vi "#1_MAV_MSG_SYS_STATUS_DECODE.vi"(11 "mavlink_payload":u8[](array[numeric])) -> (3 "SYS_STATUS":T1)   [LabVIEW 2023]
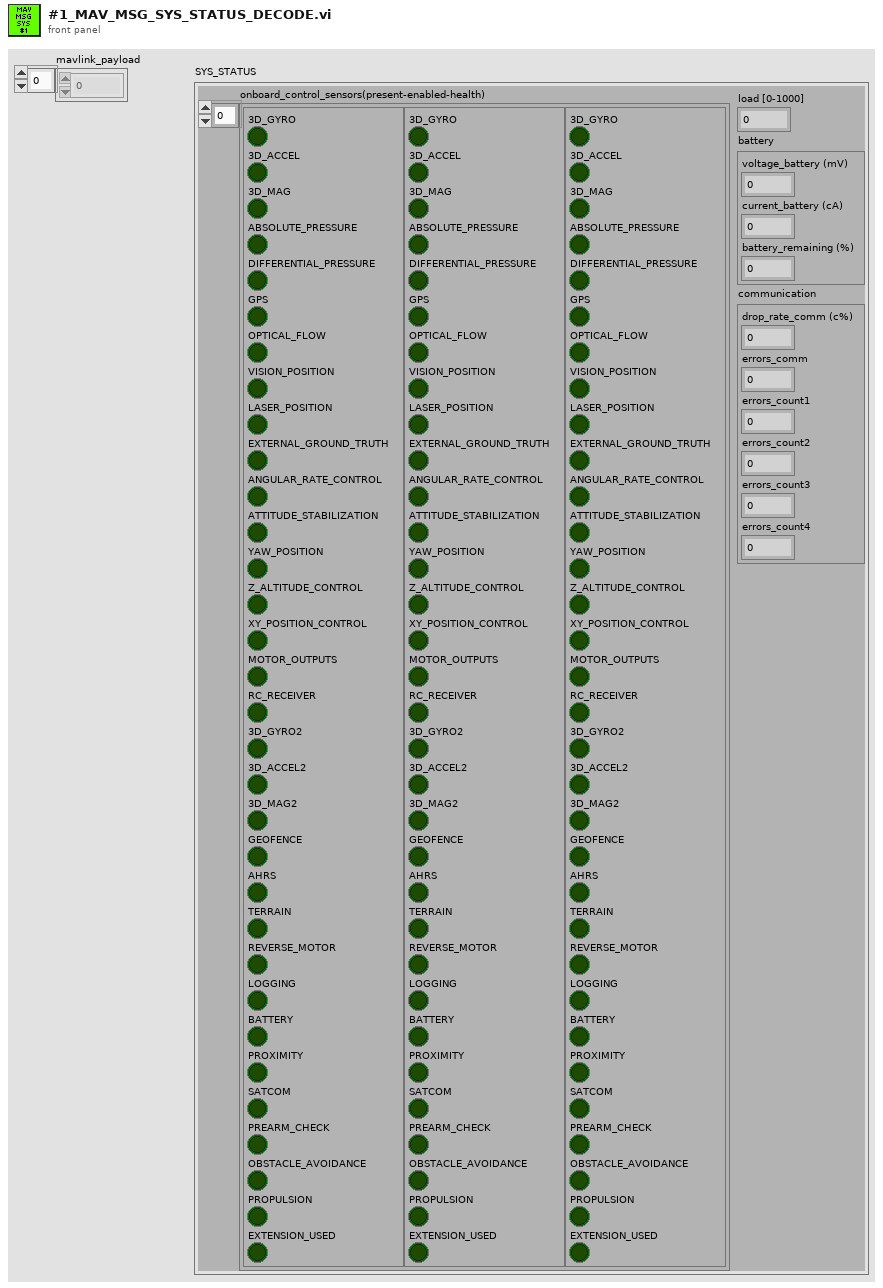
[diagram p1: front panel]
types:
  T1 = cluster{"onboard_control_sensors(present-enabled-health)":cluster{"3D_GYRO":bool, "3D_ACCEL":bool, "3D_MAG":bool, "ABSOLUTE_PRESSURE":bool, "DIFFERENTIAL_PRESSURE":bool, "GPS":bool, "OPTICAL_FLOW":bool, "VISION_POSITION":bool, "LASER_POSITION":bool, "EXTERNAL_GROUND_TRUTH":bool, "ANGULAR_RATE_CONTROL":bool, "ATTITUDE_STABILIZATION":bool, "YAW_POSITION":bool, "Z_ALTITUDE_CONTROL":bool, "XY_POSITION_CONTROL":bool, "MOTOR_OUTPUTS":bool, "RC_RECEIVER":bool, "3D_GYRO2":bool, "3D_ACCEL2":bool, "3D_MAG2":bool, "GEOFENCE":bool, "AHRS":bool, "TERRAIN":bool, "REVERSE_MOTOR":bool, "LOGGING":bool, "BATTERY":bool, "PROXIMITY":bool, "SATCOM":bool, "PREARM_CHECK":bool, "OBSTACLE_AVOIDANCE":bool, "PROPULSION":bool, "EXTENSION_USED":bool}[], "load [0-1000]":u16, "battery":cluster{"voltage_battery (mV)":u16, "current_battery (cA)":i16, "battery_remaining (%)":i8}, "communication":cluster{"drop_rate_comm (c%)":u16, "errors_comm":u16, "errors_count1":u16, "errors_count2":u16, "errors_count3":u16, "errors_count4":u16}}
  T2 = cluster{"drop_rate_comm (c%)":u16, "errors_comm":u16, "errors_count1":u16, "errors_count2":u16, "errors_count3":u16, "errors_count4":u16}
  T3 = cluster{"voltage_battery (mV)":u16, "current_battery (cA)":i16, "battery_remaining (%)":i8}
  T4 = cluster{"3D_GYRO":bool, "3D_ACCEL":bool, "3D_MAG":bool, "ABSOLUTE_PRESSURE":bool, "DIFFERENTIAL_PRESSURE":bool, "GPS":bool, "OPTICAL_FLOW":bool, "VISION_POSITION":bool, "LASER_POSITION":bool, "EXTERNAL_GROUND_TRUTH":bool, "ANGULAR_RATE_CONTROL":bool, "ATTITUDE_STABILIZATION":bool, "YAW_POSITION":bool, "Z_ALTITUDE_CONTROL":bool, "XY_POSITION_CONTROL":bool, "MOTOR_OUTPUTS":bool, "RC_RECEIVER":bool, "3D_GYRO2":bool, "3D_ACCEL2":bool, "3D_MAG2":bool, "GEOFENCE":bool, "AHRS":bool, "TERRAIN":bool, "REVERSE_MOTOR":bool, "LOGGING":bool, "BATTERY":bool, "PROXIMITY":bool, "SATCOM":bool, "PREARM_CHECK":bool, "OBSTACLE_AVOIDANCE":bool, "PROPULSION":bool, "EXTENSION_USED":bool}[]
  T5 = cluster{"Boolean array[0]":bool, "Boolean array[1]":bool, "Boolean array[2]":bool, "Boolean array[3]":bool, "Boolean array[4]":bool, "Boolean array[5]":bool, "Boolean array[6]":bool, "Boolean array[7]":bool, "Boolean array[8]":bool, "Boolean array[9]":bool, "Boolean array[10]":bool, "Boolean array[11]":bool, "Boolean array[12]":bool, "Boolean array[13]":bool, "Boolean array[14]":bool, "Boolean array[15]":bool, "Boolean array[16]":bool, "Boolean array[17]":bool, "Boolean array[18]":bool, "Boolean array[19]":bool, "Boolean array[20]":bool, "Boolean array[21]":bool, "Boolean array[22]":bool, "Boolean array[23]":bool, "Boolean array[24]":bool, "Boolean array[25]":bool, "Boolean array[26]":bool, "Boolean array[27]":bool, "Boolean array[28]":bool, "Boolean array[29]":bool, "Boolean array[30]":bool, "Boolean array[31]":bool}
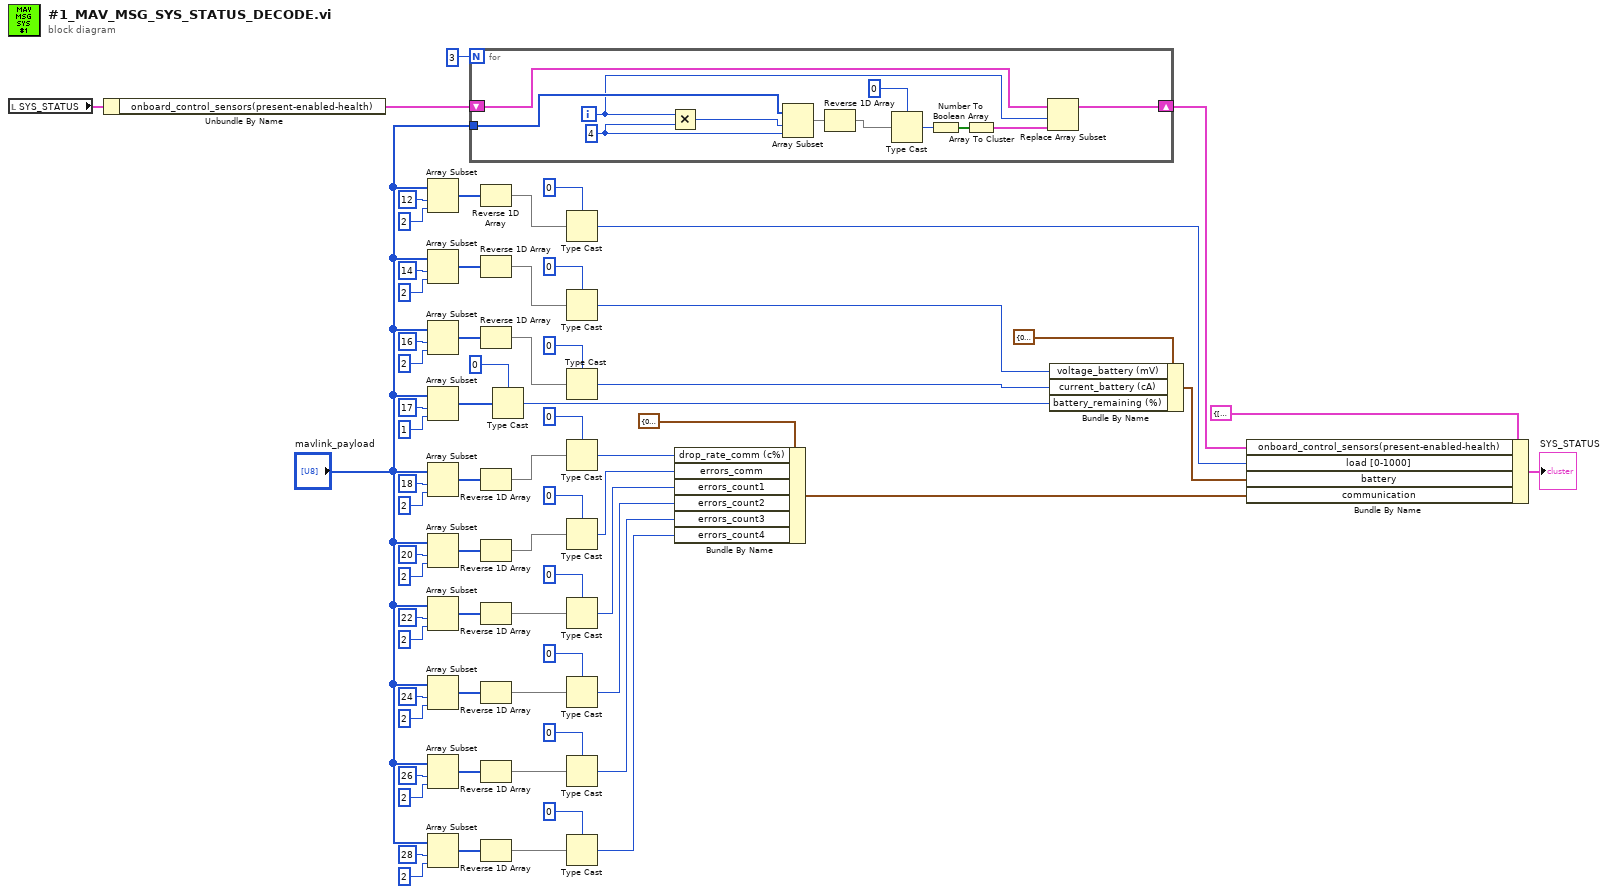
[diagram p0: block diagram]
diagram:
  n1 = local read "SYS_STATUS"() -> (w63:T1)
  n2 = Unbundle By Name(w63) -> ("onboard_control_sensors(present-enabled-health)"=w62:T4)
  n3 = Array Subset(array="mavlink_payload", index=12, length=2) -> (w65:u8[])
  n4 = Array Subset(array="mavlink_payload", index=14, length=2) -> (w60:u8[])
  n5 = Array Subset(array="mavlink_payload", index=16, length=2) -> (w50:u8[])
  n6 = Array Subset(array="mavlink_payload", index=17, length=1) -> (w41:u8[])
  n7 = Array Subset(array="mavlink_payload", index=18, length=2) -> (w38:u8[])
  n8 = Array Subset(array="mavlink_payload", index=20, length=2) -> (w30:u8[])
  n9 = Array Subset(array="mavlink_payload", index=22, length=2) -> (w24:u8[])
  n10 = Array Subset(array="mavlink_payload", index=24, length=2) -> (w19:u8[])
  n11 = Array Subset(array="mavlink_payload", index=26, length=2) -> (w12:u8[])
  n12 = Array Subset(array="mavlink_payload", index=28, length=2) -> (w7:u8[])
  n13 = for {
    N: 3 -> [_]
    tunnel: "mavlink_payload" -> [w78]
    shift-right: [w77] -> w64
    shift-left: w62 -> [w76]
    i -> [w74]
    w75 = 4 ("length")
    n14 = Multiply(x=w74, y=w75) -> (x*y=w73:i32)
    n15 = Array Subset(array=w78, index=w73, length=w75) -> (w80:u8[])
    n16 = Reverse 1D Array(array=w80) -> (reversed array=w81:u8[])
    n17 = Type Cast(type=u32 0, x=w81) -> (*(type *) &x=w82:u32)
    n18 = Number To Boolean Array(number=w82) -> (Boolean array=w72:bool[])
    n19 = Array To Cluster(array=w72) -> (cluster=w71:T5)
    n20 = Replace Array Subset(array=w76, new element=w71, index=w74) -> (w77:T4)
  }
  n21 = Reverse 1D Array(array=w65) -> (reversed array=w67:u8[])
  n22 = Reverse 1D Array(array=w60) -> (reversed array=w61:u8[])
  n23 = Reverse 1D Array(array=w50) -> (reversed array=w51:u8[])
  n24 = Reverse 1D Array(array=w38) -> (reversed array=w39:u8[])
  n25 = Reverse 1D Array(array=w30) -> (reversed array=w31:u8[])
  n26 = Reverse 1D Array(array=w24) -> (reversed array=w25:u8[])
  n27 = Reverse 1D Array(array=w19) -> (reversed array=w20:u8[])
  n28 = Reverse 1D Array(array=w12) -> (reversed array=w13:u8[])
  n29 = Reverse 1D Array(array=w7) -> (reversed array=w8:u8[])
  n30 = Type Cast(type=i8 0, x=w41) -> (*(type *) &x=w40:i8)
  n31 = Type Cast(type=u16 0, x=w67) -> (*(type *) &x=w59:u16)
  n32 = Type Cast(type=u16 0, x=w61) -> (*(type *) &x=w52:u16)
  n33 = Type Cast(type=i16 0, x=w51) -> (*(type *) &x=w47:i16)
  n34 = Type Cast(type=u16 0, x=w39) -> (*(type *) &x=w32:u16)
  n35 = Type Cast(type=u16 0, x=w31) -> (*(type *) &x=w26:u16)
  n36 = Type Cast(type=u16 0, x=w25) -> (*(type *) &x=w15:u16)
  n37 = Type Cast(type=u16 0, x=w20) -> (*(type *) &x=w14:u16)
  n38 = Type Cast(type=u16 0, x=w13) -> (*(type *) &x=w2:u16)
  n39 = Type Cast(type=u16 0, x=w8) -> (*(type *) &x=w1:u16)
  n40 = Bundle By Name(cluster=T2 {"drop_rate_comm (c%)"=0, "errors_comm"=0, "errors_count1"=0, "errors_count2"=0, "errors_count3"=0, "errors_count4"=0} ("communication"), "drop_rate_comm (c%)"=w32, "errors_comm"=w26, "errors_count1"=w15, "errors_count2"=w14, "errors_count3"=w2, "errors_count4"=w1) -> (w33:T2)
  n41 = Bundle By Name(cluster=T3 {"voltage_battery (mV)"=0, "current_battery (cA)"=0, "battery_remaining (%)"=0} ("battery"), "voltage_battery (mV)"=w52, "current_battery (cA)"=w47, "battery_remaining (%)"=w40) -> (w53:T3)
  n42 = Bundle By Name(cluster=T1 {"onboard_control_sensors(present-enabled-health)"=[{"3D_GYRO"=FALSE, "3D_ACCEL"=FALSE, "3D_MAG"=FALSE, "ABSOLUTE_PRESSURE"=FALSE, "DIFFERENTIAL_PRESSURE"=FALSE, "GPS"=FALSE, "OPTICAL_FLOW"=FALSE, "VISION_POSITION"=FALSE, "LASER_POSITION"=FALSE, "EXTERNAL_GROUND_TRUTH"=FALSE, "ANGULAR_RATE_CONTROL"=FALSE, "ATTITUDE_STABILIZATION"=FALSE, "YAW_POSITION"=FALSE, "Z_ALTITUDE_CONTROL"=FALSE, "XY_POSITION_CONTROL"=FALSE, "MOTOR_OUTPUTS"=FALSE, "RC_RECEIVER"=FALSE, "3D_GYRO2"=FALSE, "3D_ACCEL2"=FALSE, "3D_MAG2"=FALSE, "GEOFENCE"=FALSE, "AHRS"=FALSE, "TERRAIN"=FALSE, "REVERSE_MOTOR"=FALSE, "LOGGING"=FALSE, "BATTERY"=FALSE, "PROXIMITY"=FALSE, "SATCOM"=FALSE, "PREARM_CHECK"=FALSE, "OBSTACLE_AVOIDANCE"=FALSE, "PROPULSION"=FALSE, "EXTENSION_USED"=FALSE}, {"3D_GYRO"=FALSE, "3D_ACCEL"=FALSE, "3D_MAG"=FALSE, "ABSOLUTE_PRESSURE"=FALSE, "DIFFERENTIAL_PRESSURE"=FALSE, "GPS"=FALSE, "OPTICAL_FLOW"=FALSE, "VISION_POSITION"=FALSE, "LASER_POSITION"=FALSE, "EXTERNAL_GROUND_TRUTH"=FALSE, "ANGULAR_RATE_CONTROL"=FALSE, "ATTITUDE_STABILIZATION"=FALSE, "YAW_POSITION"=FALSE, "Z_ALTITUDE_CONTROL"=FALSE, "XY_POSITION_CONTROL"=FALSE, "MOTOR_OUTPUTS"=FALSE, "RC_RECEIVER"=FALSE, "3D_GYRO2"=FALSE, "3D_ACCEL2"=FALSE, "3D_MAG2"=FALSE, "GEOFENCE"=FALSE, "AHRS"=FALSE, "TERRAIN"=FALSE, "REVERSE_MOTOR"=FALSE, "LOGGING"=FALSE, "BATTERY"=FALSE, "PROXIMITY"=FALSE, "SATCOM"=FALSE, "PREARM_CHECK"=FALSE, "OBSTACLE_AVOIDANCE"=FALSE, "PROPULSION"=FALSE, "EXTENSION_USED"=FALSE}, {"3D_GYRO"=FALSE, "3D_ACCEL"=FALSE, "3D_MAG"=FALSE, "ABSOLUTE_PRESSURE"=FALSE, "DIFFERENTIAL_PRESSURE"=FALSE, "GPS"=FALSE, "OPTICAL_FLOW"=FALSE, "VISION_POSITION"=FALSE, "LASER_POSITION"=FALSE, "EXTERNAL_GROUND_TRUTH"=FALSE, "ANGULAR_RATE_CONTROL"=FALSE, "ATTITUDE_STABILIZATION"=FALSE, "YAW_POSITION"=FALSE, "Z_ALTITUDE_CONTROL"=FALSE, "XY_POSITION_CONTROL"=FALSE, "MOTOR_OUTPUTS"=FALSE, "RC_RECEIVER"=FALSE, "3D_GYRO2"=FALSE, "3D_ACCEL2"=FALSE, "3D_MAG2"=FALSE, "GEOFENCE"=FALSE, "AHRS"=FALSE, "TERRAIN"=FALSE, "REVERSE_MOTOR"=FALSE, "LOGGING"=FALSE, "BATTERY"=FALSE, "PROXIMITY"=FALSE, "SATCOM"=FALSE, "PREARM_CHECK"=FALSE, "OBSTACLE_AVOIDANCE"=FALSE, "PROPULSION"=FALSE, "EXTENSION_USED"=FALSE}], "load [0-1000]"=0, "battery"={"voltage_battery (mV)"=0, "current_battery (cA)"=0, "battery_remaining (%)"=0}, "communication"={"drop_rate_comm (c%)"=0, "errors_comm"=0, "errors_count1"=0, "errors_count2"=0, "errors_count3"=0, "errors_count4"=0}} ("Sys_Status"), "onboard_control_sensors(present-enabled-health)"=w64, "load [0-1000]"=w59, "battery"=w53, "communication"=w33) -> (→"SYS_STATUS":T1)
